vi "Set Output State.vi"(8 "error in (no error)":errorcluster, 10 "Output State":bool, 11 "Evaporative Cooler":refnum<class "Evaporative Cooler.lvclass">) -> (0 "error out":errorcluster, 3 "Evaporative Cooler":refnum<class "Evaporative Cooler.lvclass">)   [LabVIEW 2025, in "Evaporative Cooler.lvlib" / "Evaporative Cooler.lvclass"]
doc: "Child classes should not need to override this method. If they do, they must invoke the Call Parent node."
uses:
  Evaporative Cooler.lvclass
  Evaporative Cooler.lvclass/Evaporative Cooler.ctl
  <vilib>/ActorFramework/Time-Delayed Send Message/Time-Delay Override Options.ctl
  <vilib>/ActorFramework/Message Enqueuer/Message Enqueuer.lvclass/Message Enqueuer.ctl
  Dual Fan/Run Fan Msg/Run Fan Msg.lvclass
  C:/Program Files/National Instruments/LabVIEW 2025/vi.lib/ActorFramework/Message/Message.lvclass
  <vilib>/ActorFramework/Message Enqueuer/Enqueue.vi
  Dual Fan/Halt Fan Msg/Halt Fan Msg.lvclass
  <vilib>/ActorFramework/Message Priority Queue/Priority Enqueue.vi
  <vilib>/ActorFramework/Actor Framework.lvlib
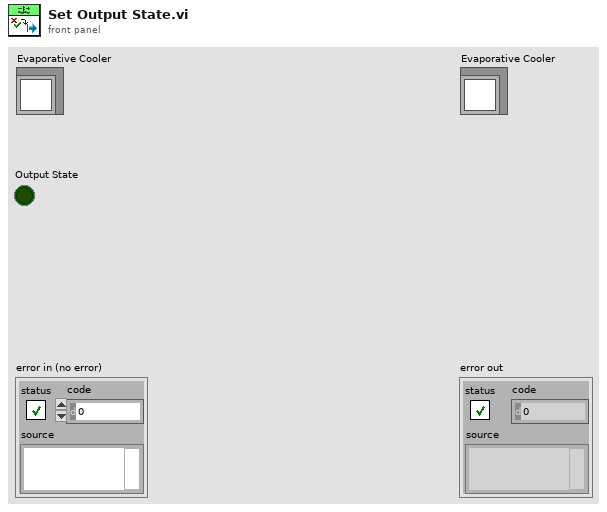
[diagram p1: front panel]
types:
  T1 = typedef "Actor Framework.lvlib/Time-Delay Override Options.ctl" = enum16{"Send next copy now", "Skip next scheduled copy", "Send next copy now and stop all further copies", "Stop all further copies"}
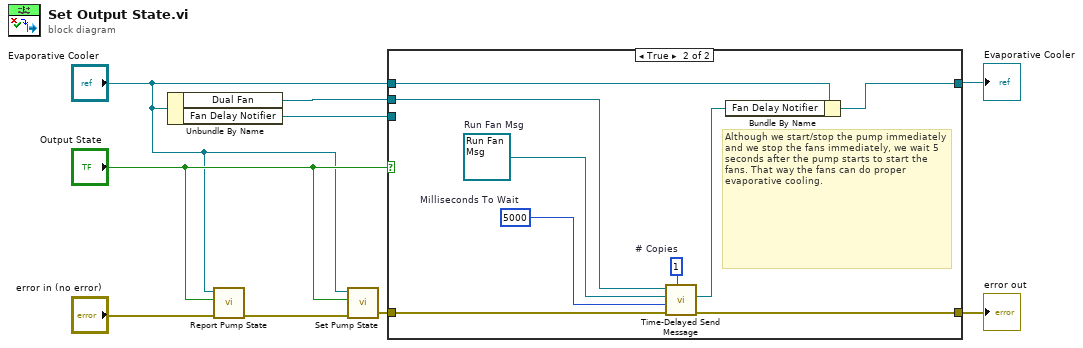
[diagram p0: block diagram]
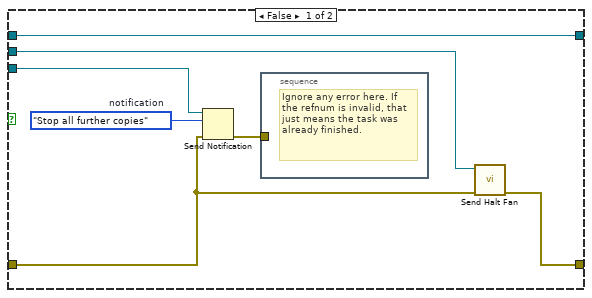
[diagram p2: hidden frame]
diagram:
  n1 = Unbundle By Name("Evaporative Cooler") -> ("Dual Fan"=w9:refnum<class "Message Enqueuer.lvclass">, "Fan Delay Notifier"=w6:refnum<notifier>)
  n2 = call "Report Pump State.vi"("error in (no error)"="error in (no error)", "Pump State"="Output State", "Evaporative Cooler in"="Evaporative Cooler") -> ("error out"=w3:errorcluster)  [unwired: 8 in]
  n3 = call-dynamic "Set Pump State.vi"("error in (no error)"=w3, "Pump State"="Output State", "Evaporative Cooler in"="Evaporative Cooler") -> ("error out"=w4:errorcluster)  [unwired: 8 in]
  n4 = case shown="True" "Output State" {
    tunnel: w4 -> [w10 w25]
    tunnel: w9 -> [w15 w19]
    tunnel: [w16 w24] -> w8
    tunnel: "Evaporative Cooler" -> [w14 w22]
    tunnel: [w14 w21] -> w7
    tunnel: w6 -> [w13 _]
    frame False {
      w12 = Time-Delay_Override_Options."Stop all further copies"  # notification
      n5 = Send Notification(notification=w12, notifier=w13, error in (no error)=w10) -> (error out=w11:errorcluster)  [unwired: 1 out]
      n6 = stacked-sequence {
        tunnel: w11 -> [_]
        frame #0 {
          # "Ignore any error here. If the refnum is invalid, that just means the task was already finished."
        }
      }
      n7 = call "Send Halt Fan.vi"("error in (no error)"=w10, "Message Enqueuer"=w15) -> ("error out"=w16:errorcluster)  [unwired: 9 in]
    }
    frame True {
      w17 = 5000  # Milliseconds To Wait
      w18 = refnum<class "Run Fan Msg.lvclass"> refnum  # Run Fan Msg
      w23 = u32 1  # # Copies
      # "Although we start/stop the pump immediately and we stop the fans immediately, we wait 5 seconds after the pump starts to start the fans. That way the fans can do proper evaporative cooling."
      n8 = call <vilib>:"Time-Delayed Send Message.vi"("# Copies (0 = infinite repeat)"=w23, "error in (no error)"=w25, "Milliseconds To Wait"=w17, "Message"=w18, "Message Enqueuer"=w19) -> ("error out"=w24:errorcluster, "Delivery Notifier"=w20:refnum<notifier>)  [unwired: 5 in]
      n9 = Bundle By Name(cluster=w22, "Fan Delay Notifier"=w20) -> (w21:refnum<class "Evaporative Cooler.lvclass">)
    }
  }
  "error out" <- w8
  "Evaporative Cooler" <- w7
